vi "Revision Query.vi"(7 "Slave Address":i32=-1 min=-1 max=30 step=1, 8 "error":errorcluster, 11 "VISA":refnum<visa-resource-name>) -> (0 "error out":errorcluster, 1 "LAN Rev":string, 2 "Control Rev":string, 3 "VISA out":refnum<visa-resource-name>, 4 "Driver Rev":string="1.03")   [LabVIEW 2025, in "TDK-Lambda GEN LAN Series.lvlib"]
doc: "Queries the instrument firmware revisions and the LavVIEW driver revision.\nControl Rev: the power supply control firmware revision\nLAN Rev: the communication interface firmware revision\n\nInstrument Driver Name: TDK-Lambda GEN LAN Series\nInstrument Manufacturer: TDK-Lambda\nInstrument Type: DC Power Supply\nSupported Models: Genesys Series, all models with LAN\nSupported Bus Types: LAN\n LAN with RS-485 Multi-Drop\n\nInstrument Driver Version: 1.03\nSupported Firmware: LAN Rev \"LAN:2.1\", \"LAN:3.1.1.9\" and above\nCreated By: Walter Heyck\nRelease Date: Nov 2019\nOriginally Developed in LabVIEW Version: LabVIEW 2018 (x64)\nOriginally Developed using VISA Version: 18.5\n\nUnsupported Instrument Features: \n- SRQ interrupt \n- Event and Enable registers\n- Self-Test\n- Calibration commands\n\nModification History: \n- Rev 1.03\n Initial release."
uses:
  <userlib>/TDK-Lambda GEN LAN Series/TDK-Lambda GEN LAN Series.lvlib
panel:
  # "TDK-Lambda Genesys \n LAN\n  DC Power Supplies"
  # "Read Revisions"
  # "(c) 2019 TDK-Lambda.  ALL RIGHTS RESERVED."
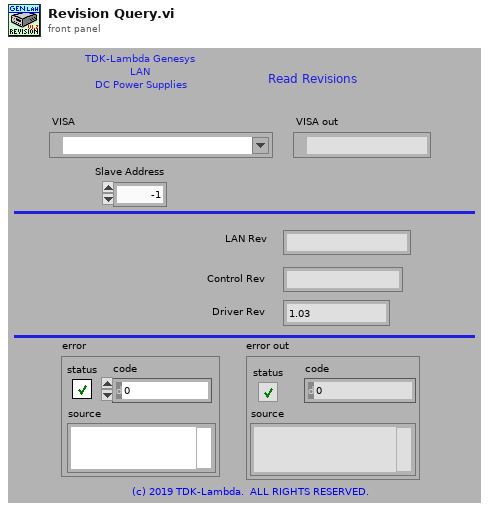
[diagram p1: front panel]
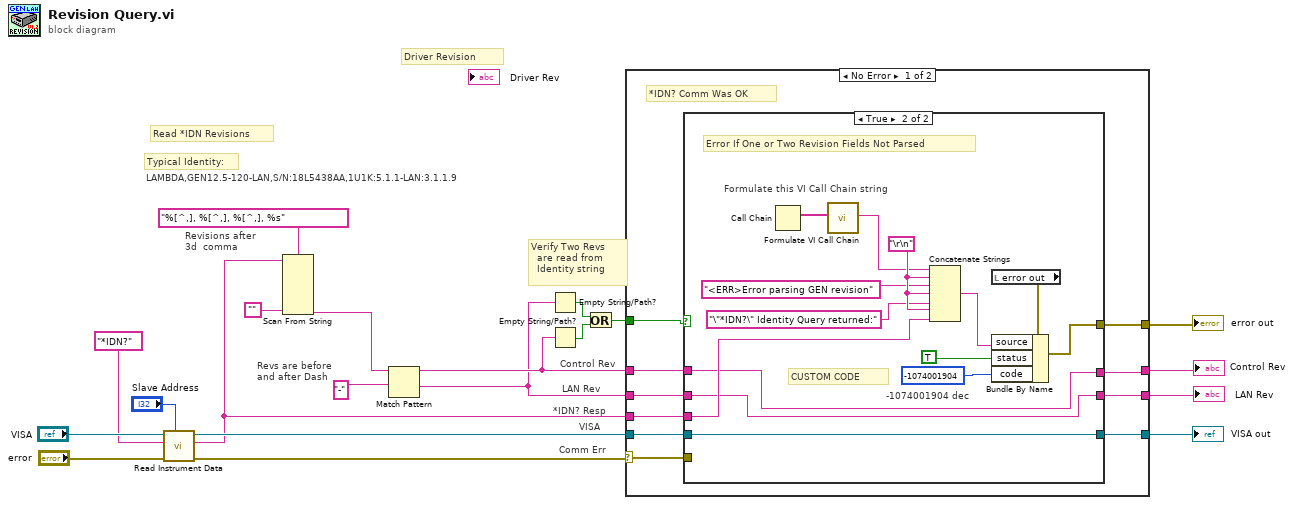
[diagram p0: block diagram]
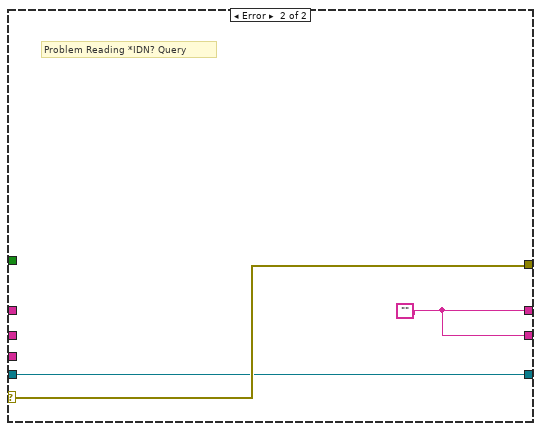
[diagram p3: hidden frame]
diagram:
  # "Revs are before\nand after Dash"
  # "Revisions after \n3d  comma"
  # "LAMBDA,GEN12.5-120-LAN,S/N:18L5438AA,1U1K:5.1.1-LAN:3.1.1.9"
  # "Comm Err"
  # "VISA"
  # "Control Rev"
  # "LAN Rev"
  # "*IDN? Resp"
  # "Verify Two Revs  \n  are read from\n  Identity string"
  # "Typical Identity:"
  # "Driver Revision"
  # "Read *IDN Revisions"
  n1 = call <userlib>:"Read Instrument Data.vi"("Slave Address"="Slave Address", "error"="error", "Query"="*IDN?", "VISA"="VISA") -> ("error out"=w15:errorcluster, "Response"=w6:string, "VISA out"=w14:refnum<visa-resource-name>)  [unwired: 4 in, 1 out]
  n2 = Scan From String(format string="%[^,], %[^,], %[^,], %s", input string=w6, default 4="") -> (output 4=w1:string)  [unwired: 8 in, 3 out]
  n3 = Match Pattern(string=w1, regular expression="-") -> (before substring=w4:string, after substring=w3:string)  [unwired: 1 in, 2 out]
  n4 = Empty String/Path?(string/path=w3) -> (empty?=w12:bool)
  n5 = Empty String/Path?(string/path=w4) -> (empty?=w11:bool)
  n6 = Or(x=w12, y=w11) -> (x .or. y?=w10:bool)
  n7 = case shown="No Error" w15 {
    selector: w15 -> [w22 w50]
    tunnel: w3 -> [w23 _]
    tunnel: w4 -> [w25 _]
    tunnel: [w26 w51] -> w17
    tunnel: [w24 w51] -> w16
    tunnel: w14 -> [w28 w49]
    tunnel: [w27 w49] -> w13
    tunnel: w10 -> [w30 _]
    tunnel: w6 -> [w29 _]
    tunnel: [w21 w50] -> w9
    frame No Error {
      # "*IDN? Comm Was OK"
      n8 = case shown="True" w30 {
        tunnel: w29 -> [_ w41]
        tunnel: w28 -> [w34 w40]
        tunnel: [w34 w40] -> w27
        tunnel: [w32 w39] -> w26
        tunnel: w25 -> [w32 w39]
        tunnel: [w33 w38] -> w24
        tunnel: w23 -> [w33 w38]
        tunnel: w22 -> [w31 _]
        tunnel: [w31 w37] -> w21
        frame False {
          # "Both Revisions Parsed \"OK\" From Identity Query"
        }
        frame True {
          w48 = "\r\n"
          # "CUSTOM CODE"
          # "-1074001904 dec"
          # "Error If One or Two Revision Fields Not Parsed"
          # "Formulate this VI Call Chain string"
          n9 = Call Chain() -> (call chain=w35:string[])
          n10 = call <userlib>:"Formulate VI Call Chain.vi"("Call Chain"=w35) -> ("String Out"=w36:string)  [unwired: 10 in]
          n11 = Concatenate Strings(w36, w48, "<ERR>Error parsing GEN revision" ("Source"), w48, "\"*IDN?\" Identity Query returned:" ("Source"), w48, w41) -> (w47:string)
          n12 = local read "error out"() -> (w46:errorcluster)
          n13 = Bundle By Name(cluster=w46, "source"=w47, "status"=TRUE, "code"=-1074001904) -> (w37:errorcluster)
        }
      }
    }
    frame Error {
      w51 = ""
      # "Problem Reading *IDN? Query"
    }
  }
  "LAN Rev" <- w16
  "VISA out" <- w13
  "error out" <- w9
  "Control Rev" <- w17
